vi "H5Oclose.vi"(6 "error in (no error)":errorcluster, 9 "Object Ref":T1) -> (0 "error out":errorcluster)   [LabVIEW 2017]
doc: "Closes an object in an HDF5 file."
uses:
  <vilib>/UPVI/lvhdf5/library.llb/HDF5 Ref.ctl
  <vilib>/UPVI/lvhdf5/hdf5.dll
panel:
  # "LVHDF5 Toolkit\nCopyright (c) 2005-2013 by Jason D. Sommerville\nCopyright (c) 2014-2015 by UPVI, LLC.\n\nThis use and distribution of this file is governed by the terms found in \nLICENSE.txt distributed with this toolkit and installed at\n <user.lib>\\_lvhdf5\\LICENSE.txt"
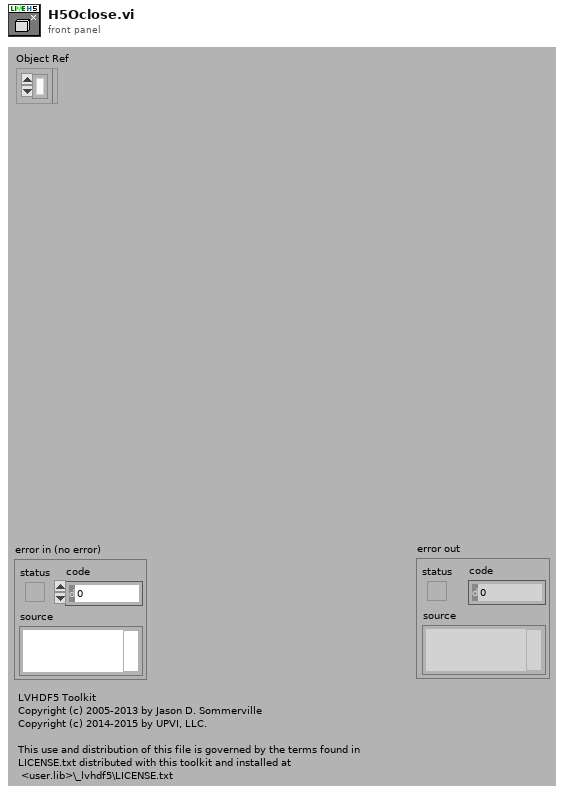
[diagram p1: front panel]
types:
  T1 = typedef "HDF5 Ref.ctl" = refnum<k1>
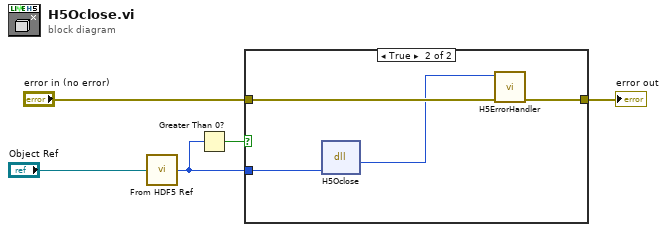
[diagram p0: block diagram]
diagram:
  n1 = call <vilib>:"From HDF5 Ref.vi"("HDF5 Ref"="Object Ref") -> ("I32"=w1:i32)
  n2 = Greater Than 0?(x=w1) -> (x > 0?=w2:bool)
  n3 = case shown="True" w2 {
    tunnel: "error in (no error)" -> [w6 w10]
    tunnel: [w6 w9] -> w4
    tunnel: w1 -> [_ w8]
    frame False {
    }
    frame True {
      n4 = dll-call lib="C:/Program Files/National Instruments/LabVIEW 2017/vi.lib/UPVI/lvhdf5/hdf5.dll" fn="H5Oclose" label="H5Oget_info"("loc_id"=w8) -> ("return type"=w7:i32)  [unwired: 4 in, 2 out]
      n5 = call <vilib>:"H5ErrorHandler.vi"("error in (no error)"=w10, "herr_t"=w7) -> ("error out"=w9:errorcluster)  [unwired: 3 in, 4 out]
    }
  }
  "error out" <- w4
